vi "test Simple Deployment.vi"(8 "error in":errorcluster, 11 "TestCase in":refnum<class "AIM Deployment.lvclass">) -> (0 "error out":errorcluster, 3 "TestCase out":refnum<class "AIM Deployment.lvclass">)   [LabVIEW 2024, in "AIM Deployment.lvclass"]
uses:
  AIM Deployment.lvclass
  AIM Deployment.lvclass/AIM Deployment.ctl
  b38e20ac-a230-4408-bc03-9f6e3cbac65d.vi
  <vilib>/addons/_JKI Toolkits/VI Tester/TestCase.llb/TestCase.lvclass
  C:/Program Files/National Instruments/LabVIEW 2024/vi.lib/addons/_JKI Toolkits/VI Tester/TestCase.llb/TestCase.lvclass
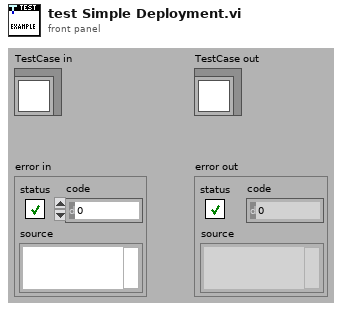
[diagram p1: front panel]
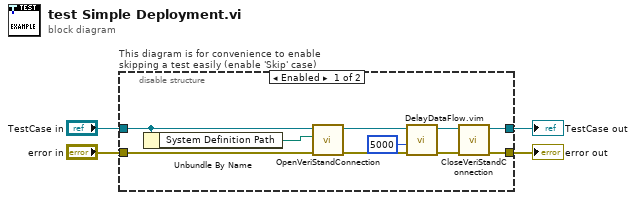
[diagram p0: block diagram]
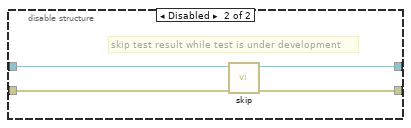
[diagram p2: hidden frame]
diagram:
  n1 = disable-structure "This diagram is for convenience to enable skipping a test easily (enable 'Skip' case)" shown="Enabled" {
    disable-tunnel: "TestCase in" -> [w5 w17]
    disable-tunnel: [w7 w15] -> w1
    disable-tunnel: [w6 w16] -> w3
    disable-tunnel: "error in" -> [w8 w14]
    frame Enabled {
      n2 = Unbundle By Name(w5) -> ("System Definition Path"=w9:path)
      n3 = call-dynamic "OpenVeriStandConnection.vi"("error in (no error)"=w8, "System Definition File"=w9, "VeriStand Test Case in"=w5) -> ("error out"=w13:errorcluster, "VeriStand Test Case out"=w10:refnum<class "AIM Deployment.lvclass">)  [unwired: 6 in, 1 out]
      n4 = call "DelayDataFlow.vim"("value in"=w13, "milliseconds to wait"=u32 5000) -> ("value out"=w11:errorcluster)  [unwired: 2 in, 1 out]
      n5 = call-dynamic "CloseVeriStandConnection.vi"("error in (no error)"=w11, "VeriStand Test Case in"=w10) -> ("error out"=w6:errorcluster, "VeriStand Test Case out"=w7:refnum<class "AIM Deployment.lvclass">)  [unwired: 8 in]
    }
    frame Disabled {
      # "skip test result while test is under development"
      n6 = call <vilib>:"skip.vi"("error in (no error)"=w14, "TestCase in"=w17) -> ("error out"=w16:errorcluster, "TestCase out"=w15:refnum<class "AIM Deployment.lvclass">)  [unwired: 8 in]
    }
  }
  "error out" <- w3
  "TestCase out" <- w1
